vi "Pressure_Transducer_Setup.vi"(1 "Setup String":string) -> (0 "Output string":string)   [LabVIEW 2020]
uses:
  File/Setup_Filetype.ctl
  Controls/ok_button.ctl
  Controls/Pressure_Units.ctl
panel:
  in  "Edit Types":bool
  in  "Pressure Units":T1
  in  "10% delta P":bool caption="100% delta P"
  in  "ID number":string
  in  "Pressure Transducer type":u16(ring) items=["FCO12 Range 0-200mmH2O", "FCO12 Range 0-20mmH2O", "FCO16 Range ±200mmH2O", "FCO16 Range ±2mmH2O", "FCO332 Range 0-0.5mmH2O", "FCO332 Range 0-200mmH2O"]
  in  "OK":T2
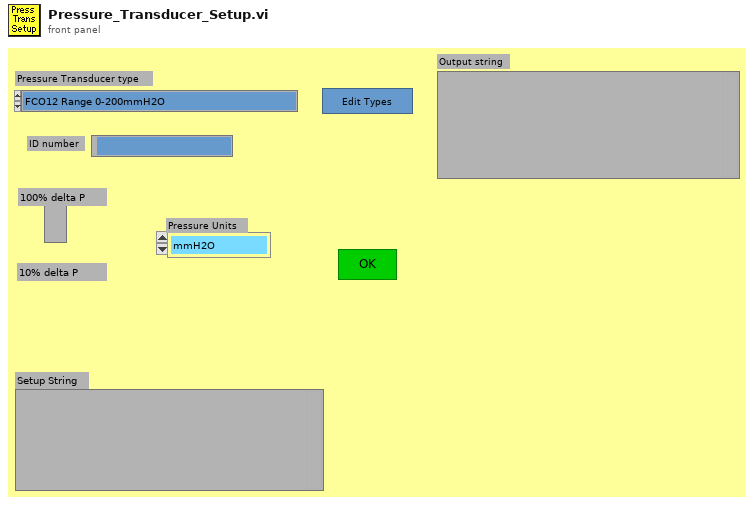
[diagram p1: front panel]
types:
  T1 = typedef "Pressure_Units.ctl" = enum16{"mmH2O", "mmHg", "Pa (N/m^2)", "mbar", "bar"}
  T2 = typedef "ok_button.ctl" = bool
  T3 = typedef "Setup_Filetype.ctl" = enum16{"Measurement Setups", "Calibration Setups", "General", "Results File Plotter Setups", "Speed Calib Tweaks"}
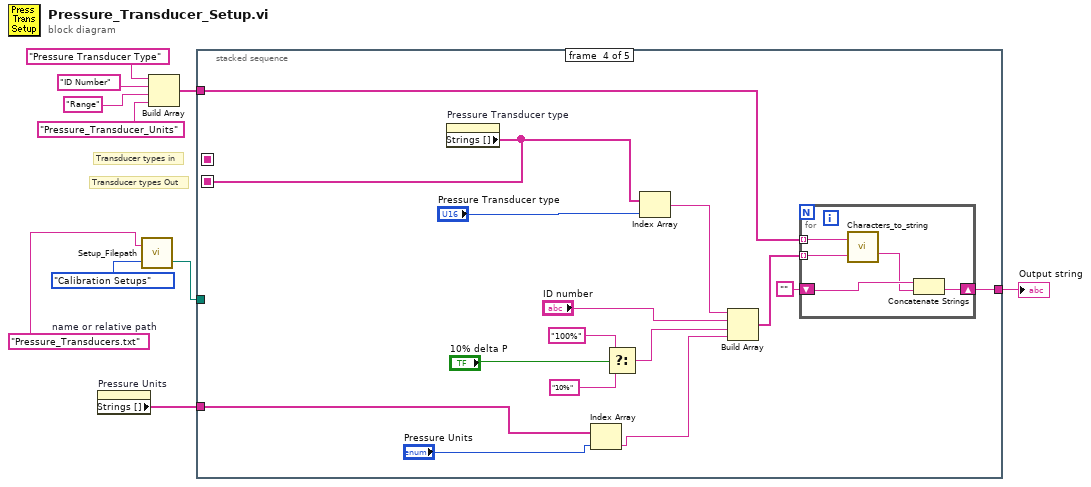
[diagram p0: block diagram]
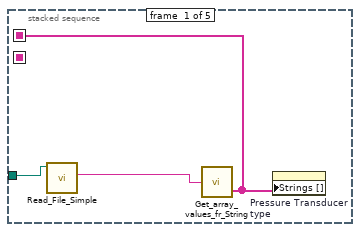
[diagram p2: hidden frame]
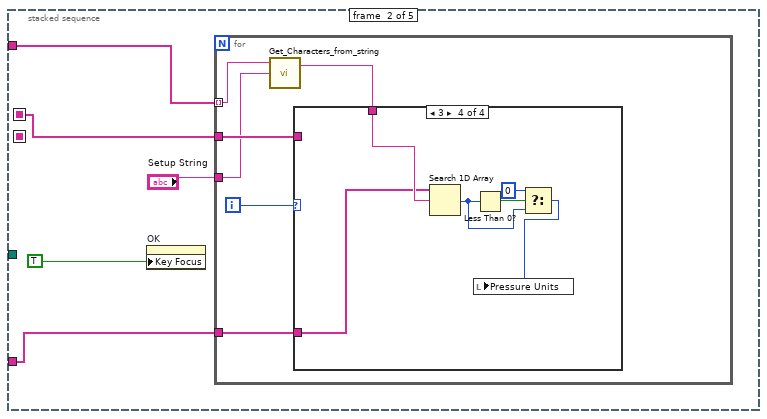
[diagram p3: hidden frame]
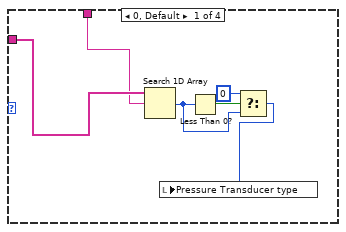
[diagram p4: hidden frame]
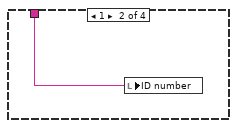
[diagram p5: hidden frame]
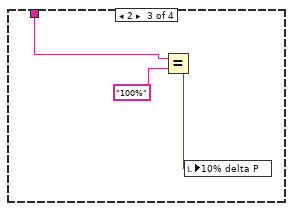
[diagram p6: hidden frame]
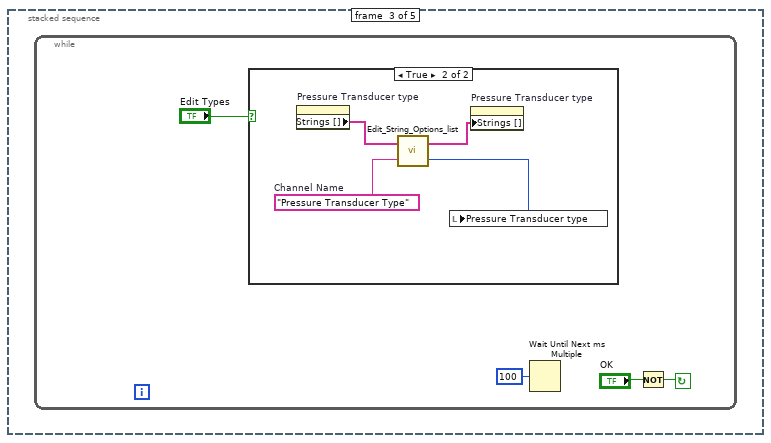
[diagram p7: hidden frame]
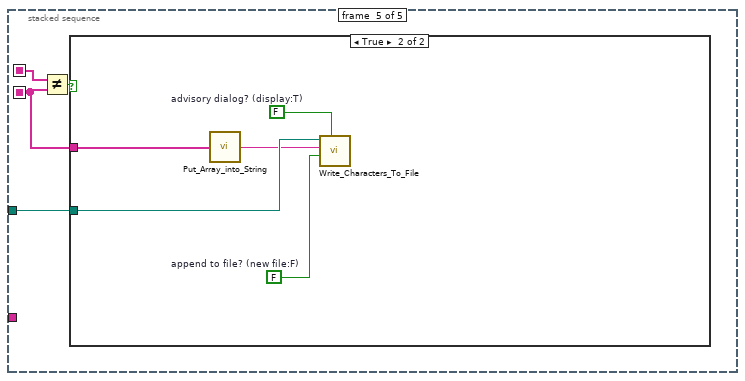
[diagram p9: hidden frame]
diagram:
  w2 = "Pressure_Transducers.txt"  # name or relative path
  # "Transducer types Out"
  # "Transducer types in"
  n1 = property on="Pressure Units" class="Enum (strict)"() -> ("Strings []"=w4:string[])  [unwired: 2 in, 2 out]
  n2 = call "Setup_Filepath.vi"("Setup File Type"=Setup_Filetype."Calibration Setups", "Filename in"=w2) -> ("Filename Out"=w1:path)  [unwired: 1 out]
  n3 = Build Array("Pressure Transducer Type", "ID Number", "Range", "Pressure_Transducer_Units") -> (w7:string[])
  n4 = stacked-sequence {
    seq-local: [w11 _ _ _ _] -> [_ w15 _ _ w72]
    seq-local: [_ _ _ w50 _] -> [_ _ _ _ w70]
    tunnel: [_ _ _ w58 _] -> w10
    tunnel: w7 -> [_ w17 _ w57 _]
    tunnel: w1 -> [w13 _ _ _ w69]
    tunnel: w4 -> [_ w14 _ w49 _]
    frame #0 {
      n5 = call "Read_File_Simple.vi"("Filename"=w13) -> ("string"=w12:string)  [unwired: 2 in, 7 out]
      n6 = call "Get_array_values_fr_String.vi"("String Value"=w12) -> ("String array"=w11:string[])  [unwired: 1 out]
      n7 = property on="Pressure Transducer type" class="Ring (strict)"("Strings []"=w11) -> ()  [unwired: 2 in, 2 out]
    }
    frame #1 {
      n8 = property on="OK" class="Bool"("Key Focus"=TRUE) -> ()  [unwired: 2 in, 2 out]
      n9 = for {
        tunnel: "Setup String" -> [w21]
        tunnel: w15 -> [w23]
        tunnel: w17 -> [w22] mode=indexing
        tunnel: w14 -> [w19]
        i -> [w24]
        n10 = call "Get_Characters_from_string.vi"("Input string"=w21, "Variable name"=w22) -> ("Value"=w20:string)  [unwired: 1 in, 1 out]
        n11 = case shown="3" w24 {
          tunnel: w23 -> [w30 _ _ _]
          tunnel: w20 -> [w29 w31 w33 w40]
          tunnel: w19 -> [_ _ _ w35]
          frame 0, Default {
            n12 = Search 1D Array(1D array=w30, element=w29) -> (index of element=w27:i32)  [unwired: 1 out]
            n13 = Less Than 0?(x=w27) -> (x < 0?=w28:bool)
            n14 = Select(t=0, s=w28, f=w27) -> (s? t:f=w25:i32)
            n15 = local write "Pressure Transducer type"(w25) -> ()
          }
          frame 1 {
            n16 = local write "ID number"(w31) -> ()
          }
          frame 2 {
            n17 = Equal?(x=w33, y="100%") -> (x = y?=w32:bool)
            n18 = local write "10% delta P"(w32) -> ()
          }
          frame 3 {
            n19 = Search 1D Array(1D array=w35, element=w40) -> (index of element=w38:i32)  [unwired: 1 out]
            n20 = Less Than 0?(x=w38) -> (x < 0?=w39:bool)
            n21 = Select(t=0, s=w39, f=w38) -> (s? t:f=w36:i32)
            n22 = local write "Pressure Units"(w36) -> ()
          }
        }
      }
    }
    frame #2 {
      n23 = while {
        stop <- w43 continue-if-true
        n24 = case shown="True" "Edit Types" {
          frame False {
          }
          frame True {
            w48 = "Pressure Transducer Type"  # Channel Name
            n25 = property on="Pressure Transducer type" class="Ring (strict)"() -> ("Strings []"=w45:string[])  [unwired: 2 in, 2 out]
            n26 = call "Edit_String_Options_list.vi"("Channel Name"=w48, "String array"=w45) -> ("New Selection Index"=w46:i32, "String array Out"=w47:string[])
            n27 = local write "Pressure Transducer type"(w46) -> ()
            n28 = property on="Pressure Transducer type" class="Ring (strict)"("Strings []"=w47) -> ()  [unwired: 2 in, 2 out]
          }
        }
        n29 = Wait Until Next ms Multiple(millisecond multiple=u32 100) -> ()  [unwired: 1 out]
        n30 = Not(x="OK") -> (.not. x?=w43:T2)
      }
    }
    frame #3 {
      n31 = property on="Pressure Transducer type" class="Ring (strict)"() -> ("Strings []"=w50:string[])  [unwired: 2 in, 2 out]
      n32 = Index Array(array=w49, index="Pressure Units") -> (element=w51:string)
      n33 = Select(t="100%", s="10% delta P", f="10%") -> (s? t:f=w56:string)
      n34 = Index Array(array=w50, index="Pressure Transducer type") -> (element=w61:string)
      n35 = Build Array(w61, "ID number", w56, w51) -> (w60:string[])
      n36 = for {
        shift-right: [w64] -> w58
        shift-left: "" -> [w66]
        tunnel: w57 -> [w68] mode=indexing
        tunnel: w60 -> [w67] mode=indexing
        n37 = call "Characters_to_string.vi"("Characters to write"=w67, "Label for characters"=w68) -> ("Output string"=w65:string)  [unwired: 1 in]
        n38 = Concatenate Strings(w66, w65) -> (w64:string)
      }
    }
    frame #4 {
      n39 = Not Equal?(x=w72, y=w70) -> (x != y?=w71:bool)
      n40 = case shown="True" w71 {
        tunnel: w70 -> [_ w77]
        tunnel: w69 -> [_ w76]
        frame False {
        }
        frame True {
          w73 = FALSE  # append to file? (new file:F)
          w74 = FALSE  # advisory dialog? (display:T)
          n41 = call "Put_Array_into_String.vi"("String array"=w77) -> ("String Value"=w75:string)
          n42 = call "Write_Characters_To_File.vi"("file path (dialog if empty)"=w76, "advisory dialog? (display:T)"=w74, "character string"=w75, "append to file? (new file:F)"=w73) -> ()  [unwired: 1 in, 4 out]
        }
      }
    }
  }
  "Output string" <- w10
